vi "myRIO_BRig_RT_dataMTrig_Audio_c__R.vi"() -> (2 "output_Audio_c__R":i32)   [LabVIEW 2014]
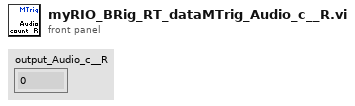
[diagram p1: front panel]
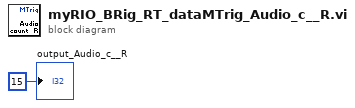
[diagram p0: block diagram]
diagram:
  "output_Audio_c__R" <- 15 ("output_iBlock")
